vi "Actor Core.vi"(8 "error in":errorcluster, 11 "Example Actor in":refnum<class "Example Actor.lvclass">) -> (0 "error out":errorcluster, 3 "Actor out":refnum<class "Actor.lvclass">)   [LabVIEW 2016, in "Example Actor.lvlib" / "Example Actor.lvclass"]
doc: "(<B>Filename</B>: Actor Framework.lvlib:Actor.lvclass:Actor Core.vi)\n\nReceives messages to the actor, reacts to them, and initiates any error handling that may shut the actor down.\n\nDescendant classes may override this VI to append parallel tasks for the actor to complete while it handles messages. Overrides use the Call Parent Method node."
uses:
  Example Actor.lvclass
  C:/Program Files (x86)/National Instruments/LabVIEW 2016/vi.lib/ActorFramework/Actor/Actor.lvclass
  <vilib>/ActorFramework/Actor/Actor.lvclass
  Iterator Settings.ctl
  Iterator Actor/Iterator Actor/Stop Condition.ctl
  Iterator Actor/Iterator Actor/Iterator Actor.lvclass
  Example Actor.lvclass/Example Actor.ctl
  <vilib>/ActorFramework/Actor/Actor.lvclass/Actor.ctl
  <vilib>/ActorFramework/Message Enqueuer/Message Enqueuer.lvclass/Message Enqueuer.ctl
  Example Actor Messages/Pre Iterate Reply Msg/Pre Iterate Reply Msg.lvclass
  C:/Project/Shared Libraries/Iterator Actor/Iterator Actor/Iterator Actor Abstract Messages/Iterator Reply Msg/Iterator Reply Msg.lvclass
  Example Actor Messages/Iterate Reply Msg/Iterate Reply Msg.lvclass
  Example Actor Messages/Post Iterate Reply Msg/Post Iterate Reply Msg.lvclass
  Example Actor Messages/Update Error Msg/Update Error Msg.lvclass
  C:/Project/Shared Libraries/Iterator Actor/Iterator Actor/Iterator Actor Abstract Messages/Iterator Report Error Msg/Iterator Report Error Msg.lvclass
  Iterator Actor/Iterator Actor/Iterator Settings.ctl
  Iterator Actor/Iterator Actor Abstract Messages/Iterator Reply Msg/Iterator Reply Msg.lvclass
  Iterator Actor/Iterator Actor Abstract Messages/Iterator Report Error Msg/Iterator Report Error Msg.lvclass
  <vilib>/ActorFramework/Message Enqueuer/Init from Existing Queue.vi
  <vilib>/ActorFramework/Message Enqueuer/Enqueue.vi
  <vilib>/ActorFramework/Stop Msg/Stop Msg.lvclass
  C:/Program Files (x86)/National Instruments/LabVIEW 2016/vi.lib/ActorFramework/Message/Message.lvclass
  <vilib>/ActorFramework/Message Priority Queue/Priority Enqueue.vi
  <vilib>/ActorFramework/Message Enqueuer/Message Enqueuer.lvclass
  Example Actor Messages/Write Ready for iterations Msg/Write Ready for iterations Msg.lvclass
  Iterator Actor/Iterator Actor Messages/Write Settings Msg/Write Settings Msg.lvclass
  Iterator Actor/Iterator Actor Messages/Start Iterations Msg/Start Iterations Msg.lvclass
  Iterator Actor/Iterator Actor Messages/Stop Iterations Msg/Stop Iterations Msg.lvclass
panel:
  out "Stopped by the Caller":bool
  out "Iterator error":errorcluster
  in  "Iterator Settings":T1={"Prepare timeout (ms)"=1000, "Iterate timeout (ms)"=1000, "Conclude timeout (ms)"=1000, "Iterate period (ms)"=1000, "Stop Condition"=enum."None", "Iterations"=5, "Time before stop (ms)"=3000}
  out "Post Iterate":bool
  out "Pre Iterate":bool
  in  "exit":bool
  out "Iterate":bool
  in  "stop iterations":bool
  in  "start iterations":bool
  in  "Ready for iterations":bool
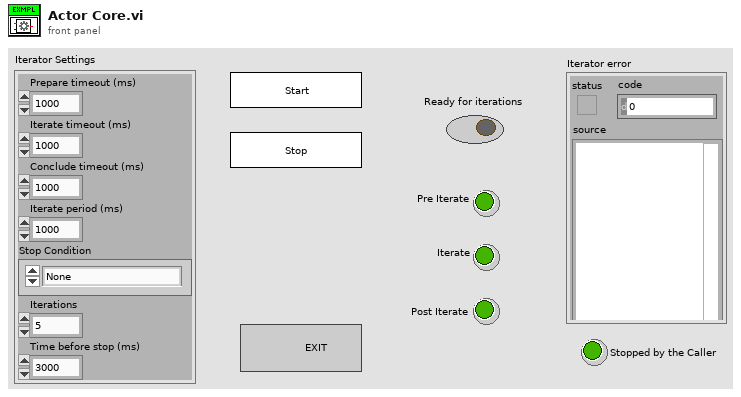
[diagram p1: front panel]
types:
  T1 = typedef "Example Actor.lvlib/Example Actor.lvclass/Iterator Settings.ctl" = cluster{"Prepare timeout (ms)":i32, "Iterate timeout (ms)":i32, "Conclude timeout (ms)":i32, "Iterate period (ms)":i32, "Stop Condition":T2, "Iterations":i32, "Time before stop (ms)":i32}
  T2 = typedef "Iterator Actor.lvlib/Iterator Actor.lvclass/Stop Condition.ctl" = enum16{"None", "Number of iterations", "Time elapsed", "Iteration result"}
  T3 = typedef "Iterator Actor.lvlib/Iterator Actor.lvclass/Iterator Settings.ctl" = cluster{"Prepare timeout (ms)":i32, "Iterate timeout (ms)":i32, "Conclude timeout (ms)":i32, "Iterate period (ms)":i32, "Number of iterations":i32, "Stop Condition":T2, "Time before stop (ms)":i32, "Prepare Msg":refnum<class "Iterator Reply Msg.lvclass">, "Iterate Msg":refnum<class "Iterator Reply Msg.lvclass">, "Conclude Msg":refnum<class "Iterator Reply Msg.lvclass">, "Error Handler":refnum<class "Iterator Report Error Msg.lvclass">}
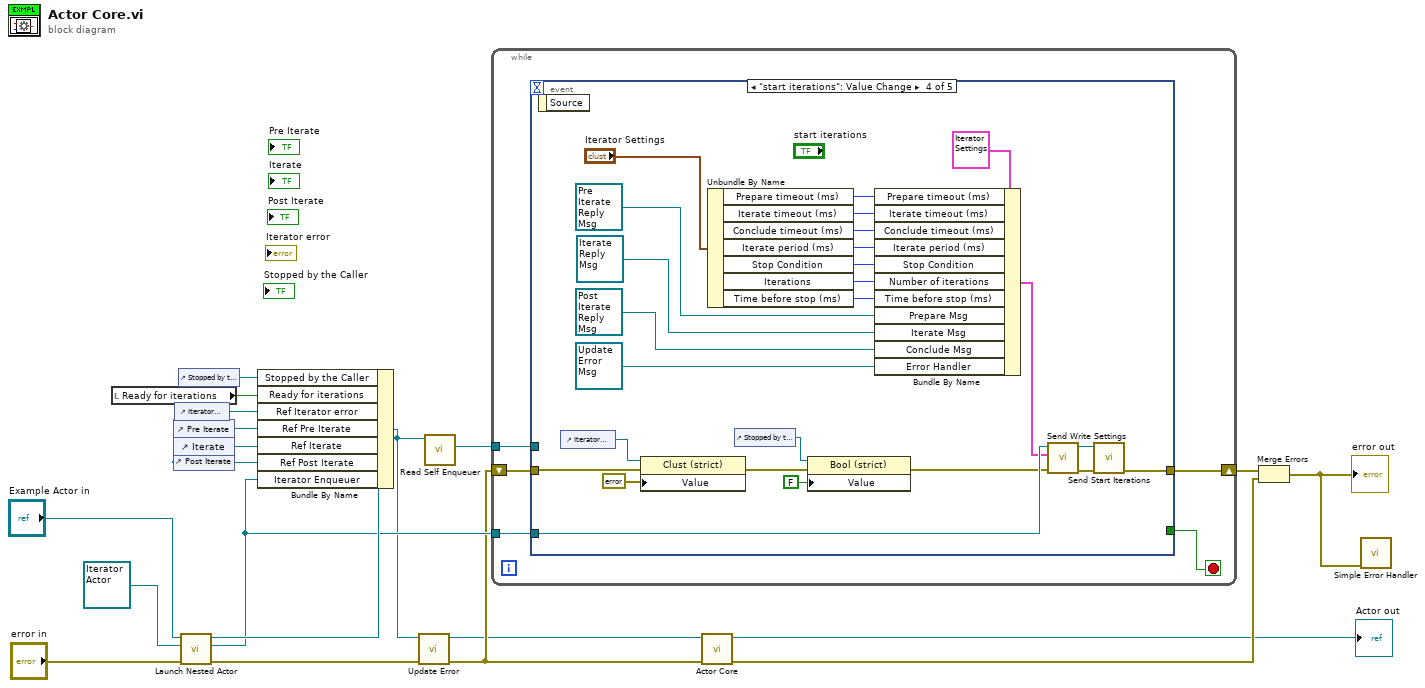
[diagram p0: block diagram]
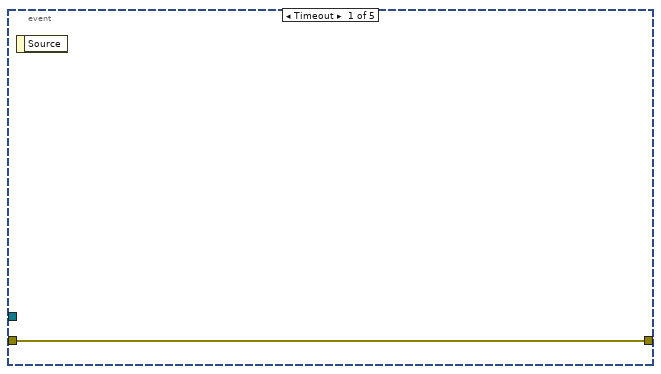
[diagram p2: hidden frame]
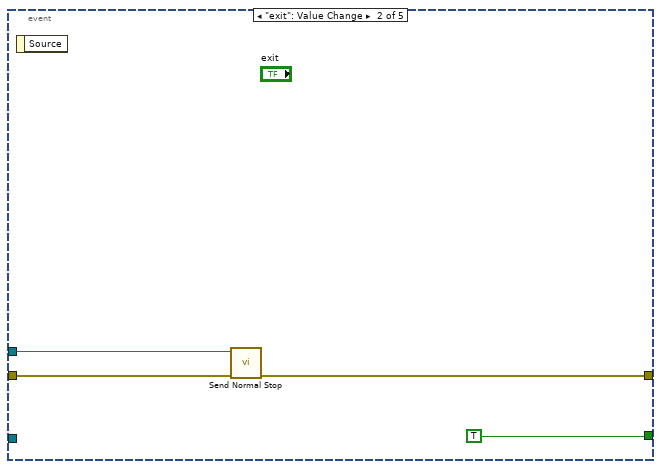
[diagram p3: hidden frame]
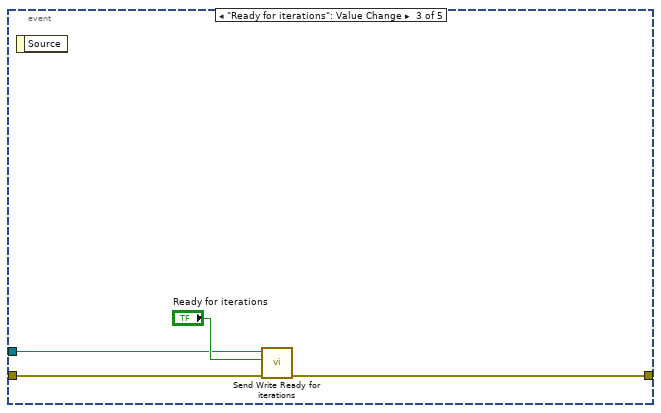
[diagram p4: hidden frame]
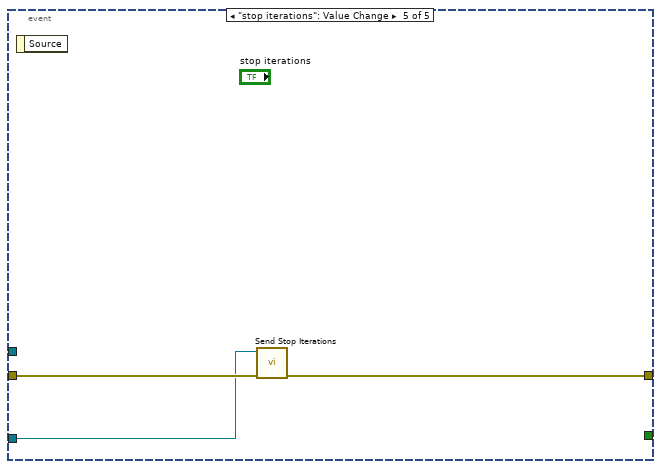
[diagram p5: hidden frame]
diagram:
  n1 = local read "Ready for iterations"() -> (w9:bool)
  n2 = control-ref of="Pre Iterate"() -> (w16:refnum<vi>)
  n3 = control-ref of="Iterate"() -> (w15:refnum<vi>)
  n4 = control-ref of="Post Iterate"() -> (w14:refnum<vi>)
  n5 = control-ref of="Iterator error"() -> (w7:refnum<vi>)
  n6 = control-ref of="Stopped by the Caller"() -> (w1:refnum<vi>)
  n7 = call <vilib>:"Launch Nested Actor.vi"("error in (no error)"="error in", "Nested Actor"=refnum<class "Iterator Actor.lvclass"> refnum ("Iterator Actor 2.lvlib:Iterator Actor 2.lvclass"), "Caller Actor in"="Example Actor in") -> ("error out"=w6:errorcluster, "Nested Actor's Enqueuer"=w10:refnum<class "Message Enqueuer.lvclass">, "Caller Actor out"=w11:refnum<class "Example Actor.lvclass">)  [unwired: 6 in]
  n8 = Bundle By Name(cluster=w11, "Stopped by the Caller"=w1, "Ready for iterations"=w9, "Ref Iterator error"=w7, "Ref Pre Iterate"=w16, "Ref Iterate"=w15, "Ref Post Iterate"=w14, "Iterator Enqueuer"=w10) -> (w4:refnum<class "Example Actor.lvclass">)
  n9 = call "Update Error.vi"("error in (no error)"=w6, "Example Actor in"=w4) -> ("error out"=w5:errorcluster, "Example Actor out"=w3:refnum<class "Example Actor.lvclass">)  [unwired: 8 in]
  n10 = call <vilib>:"Read Self Enqueuer.vi"("Actor"=w4) -> ("Self Enqueuer"=w20:refnum<class "Message Enqueuer.lvclass">)  [unwired: 10 in]
  n11 = while {
    tunnel: w20 -> [w25]
    shift-right: [w24] -> w19
    shift-left: w5 -> [w23]
    tunnel: w10 -> [w21]
    stop <- w22 stop-if-true
    n12 = event shown="[3] \"start iterations\": Value Change" {
      selector: _ -> [_ _ _ _ _]
      dyn-events: _ -> [_ _ _ _ _]
      timeout: _ -> [_ _ _ _ _]
      tunnel: w25 -> [_ w30 w31 _ _]
      tunnel: [w26 w29 w32 w41 w61] -> w24
      tunnel: w23 -> [w26 w28 w34 w44 w62]
      tunnel: [_ TRUE _ _ _] -> w22
      tunnel: w21 -> [_ _ _ w58 w60]
      event Timeout {
        n13 = event-data() -> ()  [unwired: 1 in, 1 out]
      }
      event "exit": Value Change {
        n14 = event-data() -> ()  [unwired: 1 in, 1 out]
        n15 = call <vilib>:"Send Normal Stop.vi"("error in (no error)"=w28, "Message Enqueuer"=w30) -> ("error out"=w29:errorcluster)  [unwired: 9 in]
      }
      event "Ready for iterations": Value Change {
        n16 = event-data() -> ()  [unwired: 1 in, 1 out]
        n17 = call "Send Write Ready for iterations.vi"("error in (no error)"=w34, "Ready for iterations"="Ready for iterations", "Message Enqueuer in"=w31) -> ("error out"=w32:errorcluster)  [unwired: 7 in, 1 out]
      }
      event "start iterations": Value Change {
        n18 = event-data() -> ()  [unwired: 1 in, 1 out]
        n19 = control-ref of="Iterator error"() -> (w43:refnum<vi>)
        n20 = property class="Clust (strict)"(reference=w43, error in=w44, "Value"=errorcluster {"status"=FALSE, "code"=0, "source"=""}) -> (error out=w37:errorcluster)  [unwired: 1 out]
        n21 = Unbundle By Name("Iterator Settings") -> ("Prepare timeout (ms)"=w49:i32, "Iterate timeout (ms)"=w50:i32, "Conclude timeout (ms)"=w51:i32, "Iterate period (ms)"=w52:i32, "Stop Condition"=w45:T2, "Iterations"=w46:i32, "Time before stop (ms)"=w47:i32)
        n22 = control-ref of="Stopped by the Caller"() -> (w38:refnum<vi>)
        n23 = property class="Bool (strict)"(reference=w38, error in=w37, "Value"=FALSE) -> (error out=w36:errorcluster)  [unwired: 1 out]
        n24 = Bundle By Name(cluster=T3 {"Prepare timeout (ms)"=0, "Iterate timeout (ms)"=0, "Conclude timeout (ms)"=0, "Iterate period (ms)"=0, "Number of iterations"=0, "Stop Condition"=enum."None", "Time before stop (ms)"=0, "Prepare Msg"=refnum, "Iterate Msg"=refnum, "Conclude Msg"=refnum, "Error Handler"=refnum} ("Iterator Settings"), "Prepare timeout (ms)"=w49, "Iterate timeout (ms)"=w50, "Conclude timeout (ms)"=w51, "Iterate period (ms)"=w52, "Stop Condition"=w45, "Number of iterations"=w46, "Time before stop (ms)"=w47, "Prepare Msg"=refnum<class "Pre Iterate Reply Msg.lvclass"> refnum ("Example Actor.lvlib:Pre Iterate Reply Msg.lvclass"), "Iterate Msg"=refnum<class "Iterate Reply Msg.lvclass"> refnum ("Example Actor.lvlib:Iterate Reply Msg.lvclass"), "Conclude Msg"=refnum<class "Post Iterate Reply Msg.lvclass"> refnum ("Example Actor.lvlib:Post Iterate Reply Msg.lvclass"), "Error Handler"=refnum<class "Update Error Msg.lvclass"> refnum ("Example Actor.lvlib:Update Error Msg.lvclass")) -> (w48:T3)
        n25 = call "Send Write Settings.vi"("error in (no error)"=w36, "Settings"=w48, "Message Enqueuer in"=w58) -> ("error out"=w59:errorcluster, "Message Enqueuer out"=w40:refnum<class "Message Enqueuer.lvclass">)  [unwired: 7 in]
        n26 = call "Send Start Iterations.vi"("error in (no error)"=w59, "Message Enqueuer in"=w40) -> ("error out"=w41:errorcluster)  [unwired: 8 in, 1 out]
      }
      event "stop iterations": Value Change {
        n27 = event-data() -> ()  [unwired: 1 in, 1 out]
        n28 = call "Send Stop Iterations.vi"("error in (no error)"=w62, "Message Enqueuer in"=w60) -> ("error out"=w61:errorcluster)  [unwired: 8 in, 1 out]
      }
    }
  }
  n29 = call-parent "Actor Core.vi"("error in"=w5, "Actor in"=w3) -> ("error out"=w18:errorcluster, "Actor out"=→"Actor out":refnum<class "Actor.lvclass">)  [unwired: 8 in]
  n30 = Merge Errors(w19, w18) -> (w8:errorcluster)
  "error out" <- w8
  n31 = call <vilib>:"Simple Error Handler.vi"("error in (no error)"=w8) -> ()  [unwired: 4 in, 5 out]
